vi "MerweScSigPts_ComputeWeights.vi"(8 "Kappa":i32, 9 "Beta":dbl, 10 "Alpha":dbl, 11 "States":i32) -> (1 "Wc":T1, 3 "Wm":T1)   [LabVIEW 2019, in "Trajectory_Library.lvlib"]
doc: "Computes the weights for the scaled unscented Kalman filter.\n \nInputs:\n - States -- Number of states\n - Alpha -- \n - beta -- Incorporates prior knowledge of the distribution of the mean.\n - Kapa -- \n\nOutputs:\n - Wm --"
uses:
  Trajectory_Library.lvlib
  <vilib>/Analysis/Matrix/Datatypes/RealMatrix.ctl
  <vilib>/Analysis/Matrix/NI_Matrix.lvlib
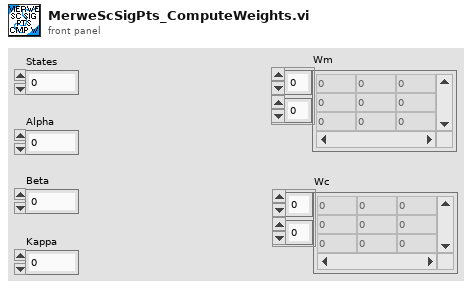
[diagram p1: front panel]
types:
  T1 = typedef "NI_Matrix.lvlib/RealMatrix.ctl" = dbl[][]
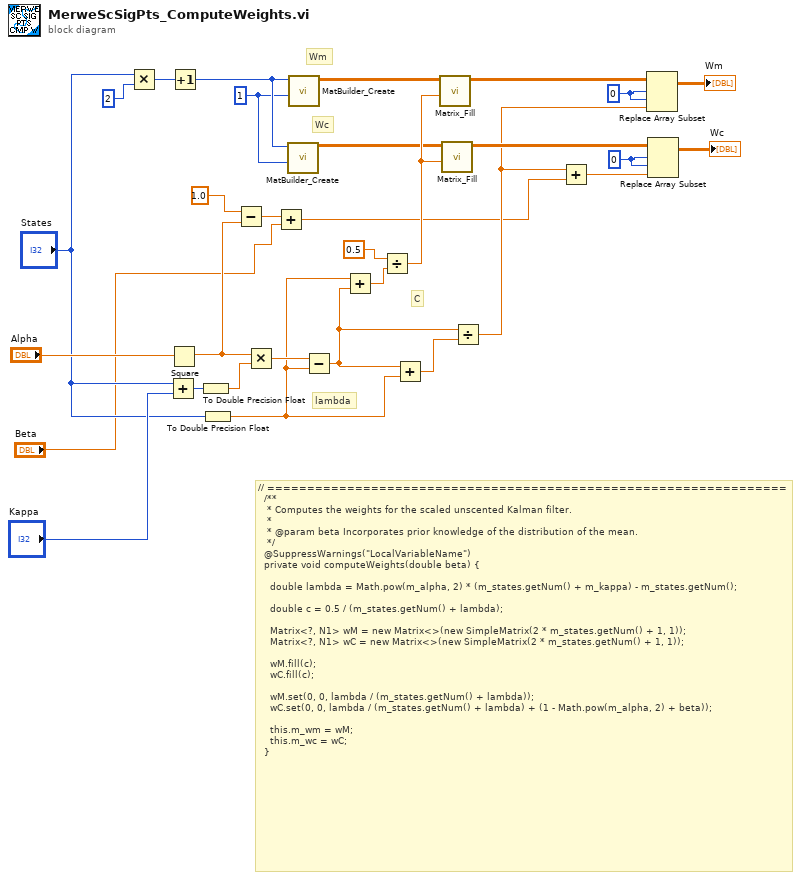
[diagram p0: block diagram]
diagram:
  w15 = 0 ("disabled index (row)")
  w16 = 0 ("disabled index (row)")
  w28 = 1 ("Columns")
  # "Wc"
  # "Wm"
  # "C"
  # "lambda"
  # "// =================================================================\n  /**\n   * Computes the weights for the scaled unscented Kalman filter.\n   *\n   * @param beta Incorporates prior knowledge of the distribution of the mean.\n   */\n  @SuppressWarnings(\"LocalVariableName\")\n  private void computeWeights(double beta) {\n\n    double lambda = Math.pow(m_alpha, 2) * (m_states.getNum() + m_kappa) - m_states.getNum();\n\n    double c = 0.5 / (m_states.getNum() + lambda);\n\n    Matrix<?, N1> wM = new Matrix<>(new SimpleMatrix(2 * m_states.getNum() + 1, 1));\n    Matrix<?, N1> wC = new Matrix<>(new SimpleMatrix(2 * m_states.getNum() + 1, 1));\n\n    wM.fill(c);\n    wC.fill(c);\n\n    wM.set(0, 0, lambda / (m_states.getNum() + lambda));\n    wC.set(0, 0, lambda / (m_states.getNum() + lambda) + (1 - Math.pow(m_alpha, 2) + beta));\n\n    this.m_wm = wM;\n    this.m_wc = wC;\n  }"
  n1 = Multiply(x="States", y=2) -> (x*y=w30:i32)
  n2 = Add(x="States", y="Kappa") -> (x+y=w25:i32)
  n3 = Square(x="Alpha") -> (x^2=w6:dbl)
  n4 = Increment(x=w30) -> (x+1=w29:i32)
  n5 = To Double Precision Float(number=w25) -> (double precision float=w23:dbl)
  n6 = To Double Precision Float(number="States") -> (double precision float=w10:dbl)
  n7 = Subtract(x=1.0, y=w6) -> (x-y=w5:dbl)
  n8 = Multiply(x=w6, y=w23) -> (x*y=w22:dbl)
  n9 = Add(x=w5, y="Beta") -> (x+y=w2:dbl)
  n10 = call "MatBuilder_Create.vi"("Columns"=w28, "Rows"=w29) -> ("output matrix"=w17:T1)  [unwired: 9 in]
  n11 = call "MatBuilder_Create.vi"("Columns"=w28, "Rows"=w29) -> ("output matrix"=w18:T1)  [unwired: 9 in]
  n12 = Subtract(x=w22, y=w10) -> (x-y=w9:dbl)
  n13 = Add(x=w10, y=w9) -> (x+y=w21:dbl)
  n14 = Divide(x=0.5, y=w21) -> (x/y=w19:dbl)
  n15 = Add(x=w9, y=w10) -> (x+y=w8:dbl)
  n16 = call "Matrix_Fill.vi"("Value"=w19, "input matrix"=w18) -> ("output matrix"=w14:T1)  [unwired: 9 in]
  n17 = call "Matrix_Fill.vi"("Value"=w19, "input matrix"=w17) -> ("output matrix"=w13:T1)  [unwired: 9 in]
  n18 = Divide(x=w9, y=w8) -> (x/y=w3:dbl)
  n19 = Add(x=w3, y=w2) -> (x+y=w1:dbl)
  n20 = Replace Array Subset(array=w14, new element=w3, index (row)=w16, index (col)=w16) -> (→"Wm":T1)
  n21 = Replace Array Subset(array=w13, new element=w1, index (row)=w15, index (col)=w15) -> (→"Wc":T1)
